vi "Timeout.vi"(8 "Start Time":u32, 11 "Time out":u32) -> (3 "Done":bool)   [LabVIEW 2014]
panel:
  # "Input the number of milliseconds to wait in Time Out.\nInput the start time into Start Time.\nWhen that many milliseconds have passed since start\ntime, done will be true."
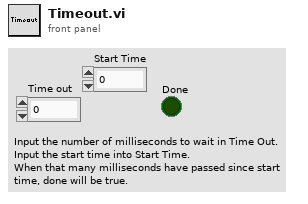
[diagram p1: front panel]
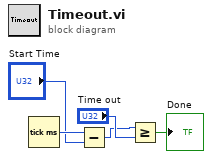
[diagram p0: block diagram]
diagram:
  n1 = Tick Count (ms)() -> (millisecond timer value=w5:u32)
  n2 = Subtract(x=w5, y="Start Time") -> (x-y=w1:u32)
  n3 = Greater Or Equal?(x=w1, y="Time out") -> (x >= y?=→"Done":bool)
